vi "OICB - Set PWM.vi"(8 "error in (no error)":errorcluster, 11 "PWM Outputs":T1) -> (0 "error out":errorcluster)   [LabVIEW 2015]
uses:
  PWM_Output_TypeDef.ctl
  <vilib>/Rock Robotics/Network Tables/NT Write Numeric Array.vi
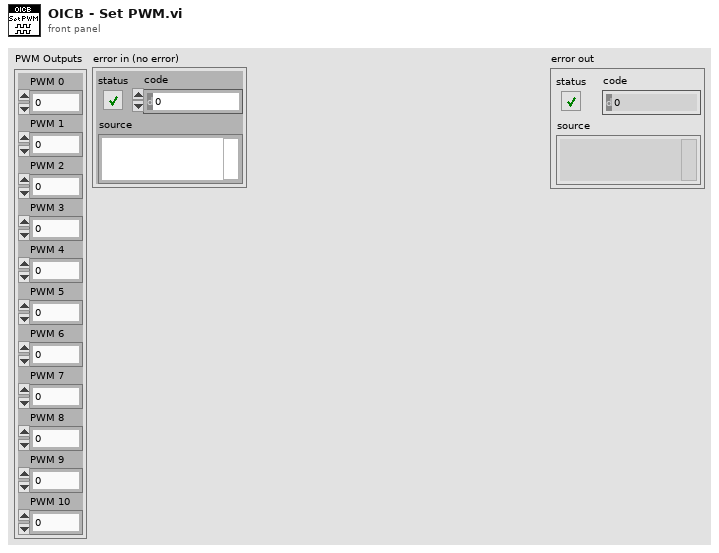
[diagram p1: front panel]
types:
  T1 = typedef "PWM_Output_TypeDef.ctl" = cluster{"PWM 0":u8, "PWM 1":u8, "PWM 2":u8, "PWM 3":u8, "PWM 4":u8, "PWM 5":u8, "PWM 6":u8, "PWM 7":u8, "PWM 8":u8, "PWM 9":u8, "PWM 10":u8}
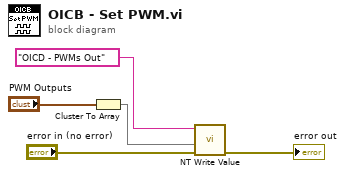
[diagram p0: block diagram]
diagram:
  n1 = Cluster To Array(cluster="PWM Outputs") -> (array=w2:u8[])
  n2 = call-poly <vilib>:"NT Write Value.vi"("error in"="error in (no error)", "Numeric Array"=w2, "Name"="OICD - PWMs Out") -> ("error out"=→"error out":errorcluster)  [unwired: 8 in]
